vi "recipeScript getTimeStamp.vi"(1 "timeFormat":timestamp) -> (0 "timeStamp":string)   [LabVIEW 2018]
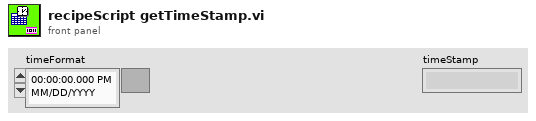
[diagram p1: front panel]
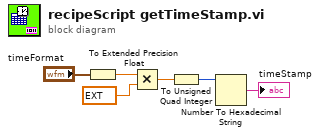
[diagram p0: block diagram]
diagram:
  n1 = To Extended Precision Float(1:"timeFormat") -> (0:w3:ext)
  n2 = Multiply(x=w3, y=ext 1000.0) -> (x*y=w5:ext)
  n3 = To Unsigned Quad Integer(1:w5) -> (0:w4:u64)
  n4 = Number To Hexadecimal String(2:w4) -> (0:→"timeStamp":string)  [unwired: 1 in]
